vi "Remove All Variable.vi"(8 "error in (no error)":errorcluster, 9 "Variable Tree":refnum<vi>, 10 "Variable Type":enum16{"Project", "Execution"}(ring), 11 "Project in":refnum<class "Project.lvclass">) -> (0 "error out":errorcluster, 3 "Project out":refnum<class "Project.lvclass">)   [LabVIEW 2015, in "Project.lvclass"]
uses:
  Project.lvclass
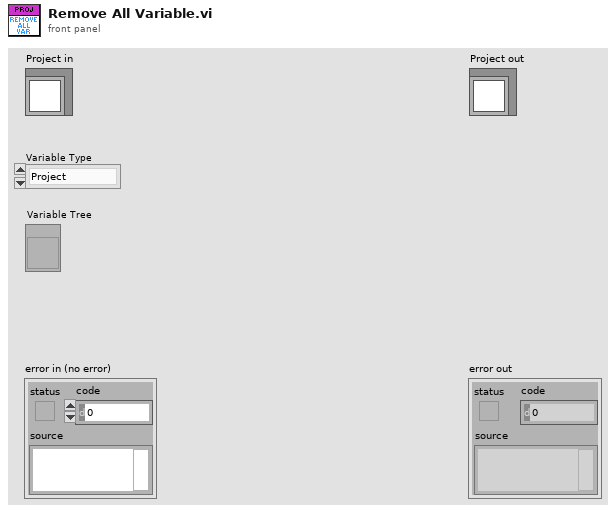
[diagram p1: front panel]
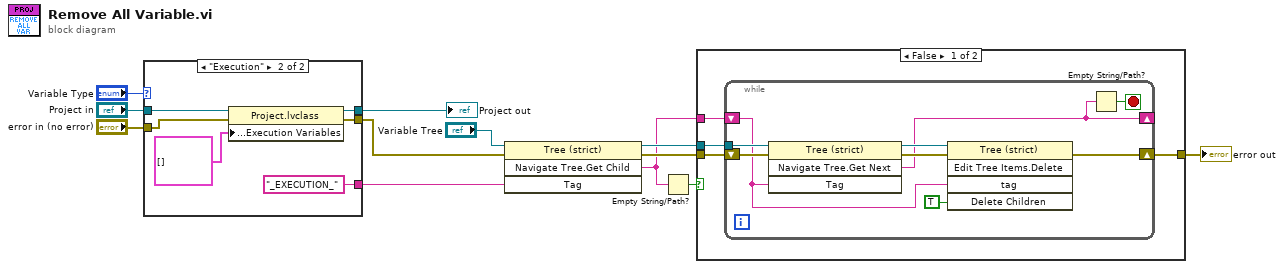
[diagram p0: block diagram]
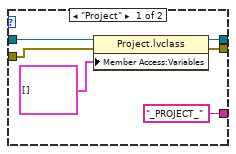
[diagram p3: hidden frame]
diagram:
  n1 = case shown="\"Execution\"" "Variable Type" {
    tunnel: "Project in" -> [w18 w24]
    tunnel: [w17 w23] -> w1
    tunnel: "error in (no error)" -> [w15 w21]
    tunnel: [w14 w20] -> w7
    tunnel: ["_PROJECT_" "_EXECUTION_"] -> w6
    frame "Project" {
      n2 = property class="Project.lvclass"(reference=w18, error in=w15, "Member Access:Variables"=cluster{"Name":string, "Value":variant}[] [] ("Execution Variables")) -> (reference out=w17:refnum<class "Project.lvclass">, error out=w14:errorcluster)
    }
    frame "Execution" {
      n3 = property class="Project.lvclass"(reference=w24, error in=w21, "Member Access:Execution Variables"=cluster{"Name":string, "Value":variant}[] [] ("Execution Variables")) -> (reference out=w23:refnum<class "Project.lvclass">, error out=w20:errorcluster)
    }
  }
  "Project out" <- w1
  n4 = invoke class="Tree (strict)" method="Navigate Tree.Get Child"(reference="Variable Tree", error in=w7, "Tag"=w6) -> (reference out=w12:refnum<vi>, error out=w4:errorcluster, "Navigate Tree:Get Child"=w3:string)  [unwired: 1 in, 1 out]
  n5 = Empty String/Path?(string/path=w3) -> (empty?=w5:bool)
  n6 = case shown="False" w5 {
    tunnel: w12 -> [w28 _]
    tunnel: w4 -> [w27 w38]
    tunnel: w3 -> [w26 _]
    tunnel: [w25 w38] -> w2
    frame False {
      n7 = while {
        tunnel: w28 -> [w37]
        shift-right: [w31] -> w25
        shift-left: w27 -> [w36]
        shift-right: [w30] -> _
        shift-left: w26 -> [w33]
        stop <- w29 stop-if-true
        n8 = invoke class="Tree (strict)" method="Navigate Tree.Get Next"(reference=w37, error in=w36, "Tag"=w33) -> (reference out=w35:refnum<vi>, error out=w34:errorcluster, "Navigate Tree:Get Next Item"=w30:string)  [unwired: 1 in, 1 out]
        n9 = invoke class="Tree (strict)" method="Edit Tree Items.Delete"(reference=w35, error in=w34, "tag"=w33, "Delete Children"=TRUE) -> (error out=w31:errorcluster)  [unwired: 1 in, 4 out]
        n10 = Empty String/Path?(string/path=w30) -> (empty?=w29:bool)
      }
    }
    frame True {
    }
  }
  "error out" <- w2
